vi "ITX Folder to HDF5.vi"(8 "error in (no error)":errorcluster, 11 "LV to ITX.lvclass":refnum<class "Data.ITX.lvclass">) -> (0 "error out":errorcluster, 3 "LV to ITX.lvclass":refnum<class "Data.ITX.lvclass">)   [LabVIEW 2016]
uses:
  Data.ITX/Data.ITX.lvclass
panel:
  in  "Folder Path":path
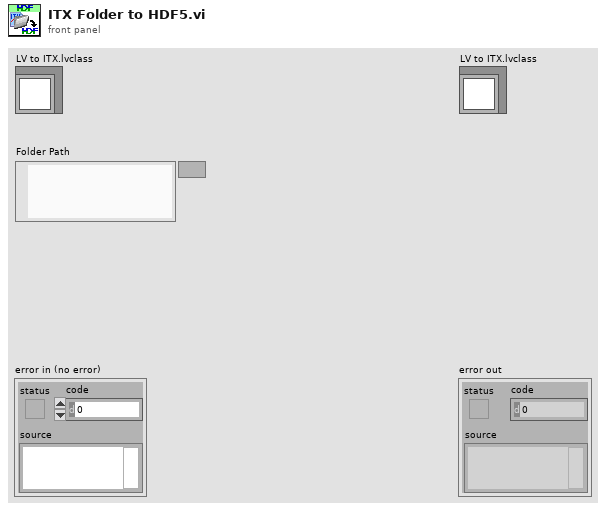
[diagram p1: front panel]
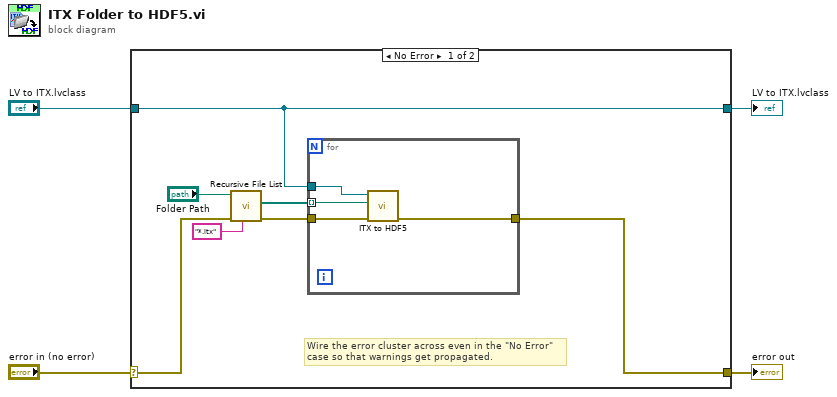
[diagram p0: block diagram]
diagram:
  n1 = case shown="No Error" "error in (no error)" {
    selector: "error in (no error)" -> [w6 w17]
    tunnel: [w5 w17] -> w3
    tunnel: [w8 w16] -> w1
    tunnel: "LV to ITX.lvclass" -> [w8 w16]
    frame No Error {
      # "Wire the error cluster across even in the \"No Error\"\ncase so that warnings get propagated."
      n2 = call <vilib>:"Recursive File List.vi"("pattern"="*.itx", "error in (no error)"=w6, "Folder Path"="Folder Path") -> ("error out"=w7:errorcluster, "All Files in Dir"=w9:path[])  [unwired: 4 in, 3 out]
      n3 = for {
        tunnel: w9 -> [w15] mode=indexing
        tunnel: w8 -> [w14]
        tunnel: w7 -> [w13]
        tunnel: [w12] -> w5
        n4 = call "ITX to HDF5.vi"("error in (no error)"=w13, "file (use dialog)"=w15, "LV to ITX.lvclass"=w14) -> ("error out"=w12:errorcluster)  [unwired: 7 in, 1 out]
      }
    }
    frame Error {
    }
  }
  "error out" <- w3
  "LV to ITX.lvclass" <- w1
